vi "SMU tester.vi"() -> ()   [LabVIEW 2021, in "Source meter.lvlib"]
uses:
  Source meter.lvlib
  ctls/SMU settings.ctl
  ctls/SMU status.ctl
  ctls/MSG to SMU.ctl
  ctls/SMU Commands.ctl
  Messenger service/MessengerLib.lvlib
panel:
  out "Event Logger":string[](array[string])
  out "data":dbl
  out "SMU status":T1 {"Measure Function" items=["Volts", "Current", "Auto Resistance", "Manual Resistance", "Digitize Voltage", "Digitize Current"]; "Source Mode" items=["Voltage", "Current"]}
  out "Last msg":timestamp
  out "Last log msg":string
  in  "VISA resource name":refnum<visa-resource-name>
  out "Waveform Chart":dbl(graph)
  in  "Measurement settings":T2={"Source Mode "=1, "Source Level"=0.001, "Source Limit"=0.1, "Measure Function"=0, "Remote sense"=FALSE, "Clear buffer?"=FALSE, "Beep"=FALSE, "High Capacity"=FALSE, "Terminals"=0, "PLCs"=1.0, "Fast measurement"=FALSE} {"Measure Function" items=["Volts", "Current", "Auto Resistance", "Manual Resistance", "Digitize Voltage", "Digitize Current"]; "Source Mode" items=["Voltage", "Current"]; "Terminals" items=["Front", "Rear"]}
  in  "Disconnect":bool
  in  "Setup measuerment":bool
  in  "Start measurment":bool
  in  "Stop measurement":bool
  in  "End":bool
  in  "Connect":bool
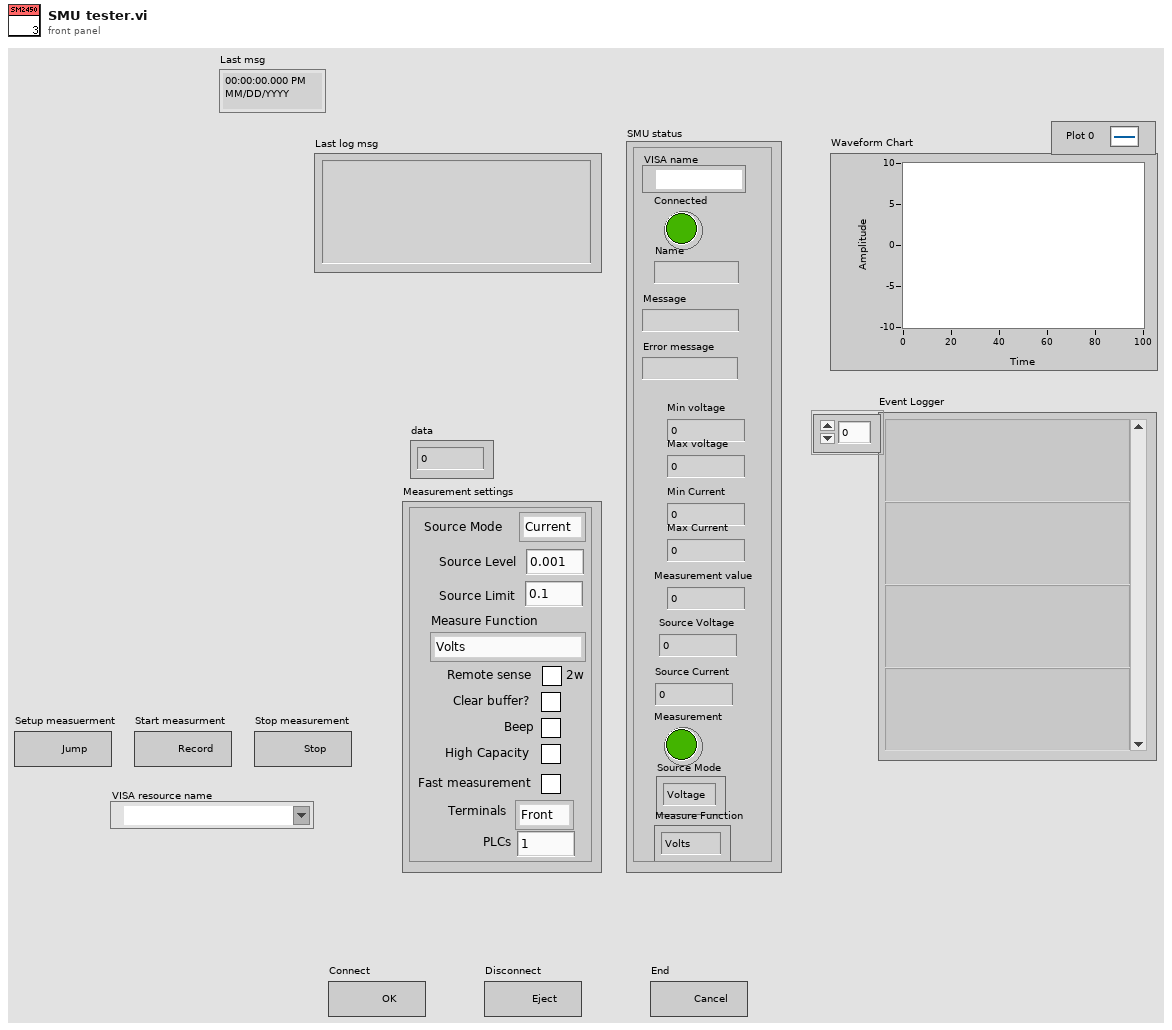
[diagram p1: front panel]
types:
  T1 = typedef "Source meter.lvlib/SMU status.ctl" = cluster{"VISA name":refnum<visa-resource-name>, "Connected":bool, "Name":string, "Message":string, "Error message":string, "Min voltage":dbl, "Max voltage":dbl, "Min Current":dbl, "Max Current":dbl, "Measurement value":dbl, "Source Voltage":dbl, "Measurement":bool, "Source Current":dbl, "Source Mode":u16, "Measure Function":u16}
  T2 = typedef "SMU settings.ctl" = cluster{"Source Mode ":u16, "Source Level":dbl, "Source Limit":dbl, "Measure Function":u16, "Remote sense":bool, "Clear buffer?":bool, "Beep":bool, "High Capacity":bool, "Terminals":u16, "PLCs":dbl, "Fast measurement":bool}
  T3 = enum16{"Initializze", "Wait for event", "Check message", "End"}
  T4 = typedef "Source meter.lvlib/MSG to SMU.ctl" = cluster{"Command":T5, "Data":variant}
  T5 = typedef "Source meter.lvlib/SMU Commands.ctl" = enum16{"Ignore", "Connect", "Update", "Set measurement", "Start measurement", "Get actual results", "Stop measurement", "Disconnect", "End"}
  T6 = typedef "MessengerLib.lvlib/MSG to TOP.ctl" = cluster{"Module":T7, "Response":string, "Data":variant, "Time":timestamp}
  T7 = typedef "Module name.ctl" = enum16{"Emty", "Magnet", "VTI", "Excitation", "Servo", "Acquisition", "Rotator", "Digitizer", "SMU2450", "Carousel", "Multimeter", "Tmp monitor", "Power monitor"}
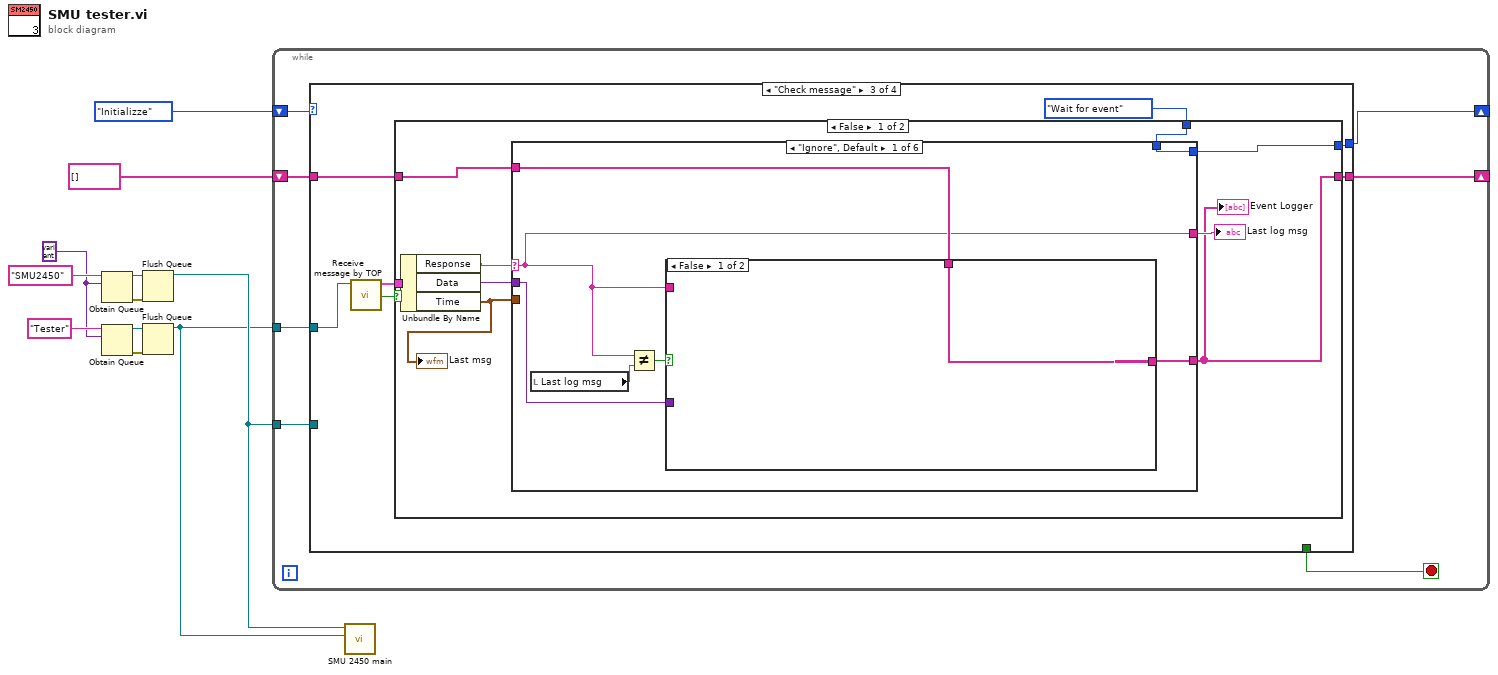
[diagram p0: block diagram]
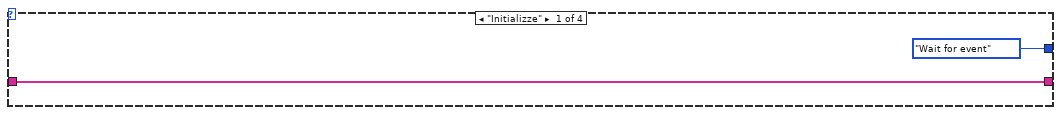
[diagram p2: hidden frame]
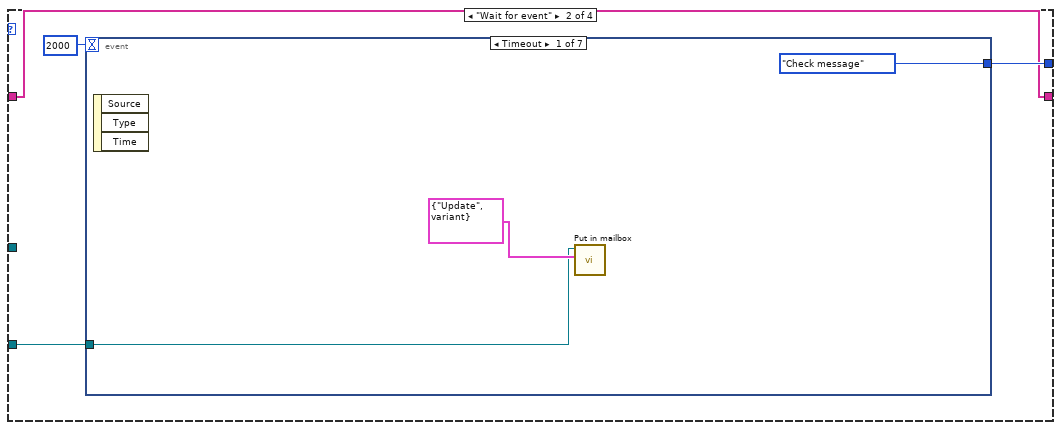
[diagram p3: hidden frame]
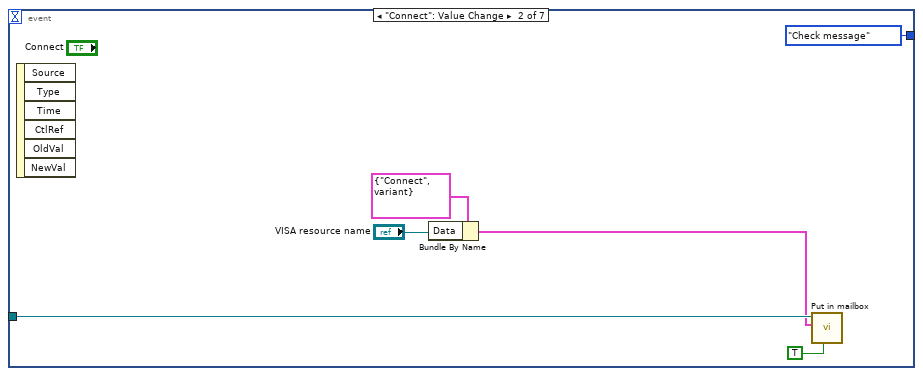
[diagram p4: hidden frame]
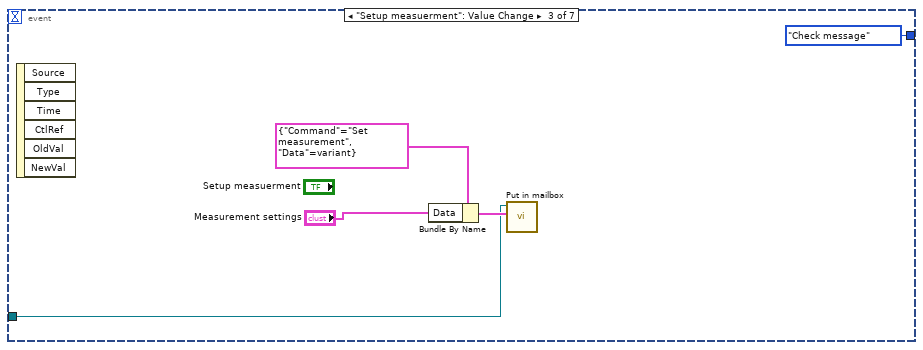
[diagram p5: hidden frame]
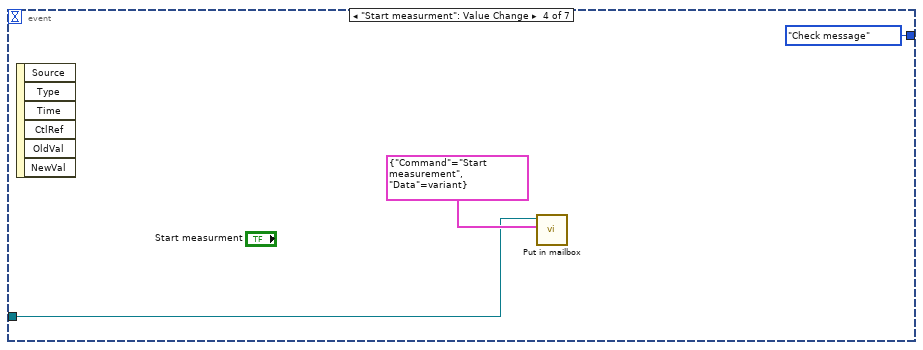
[diagram p6: hidden frame]
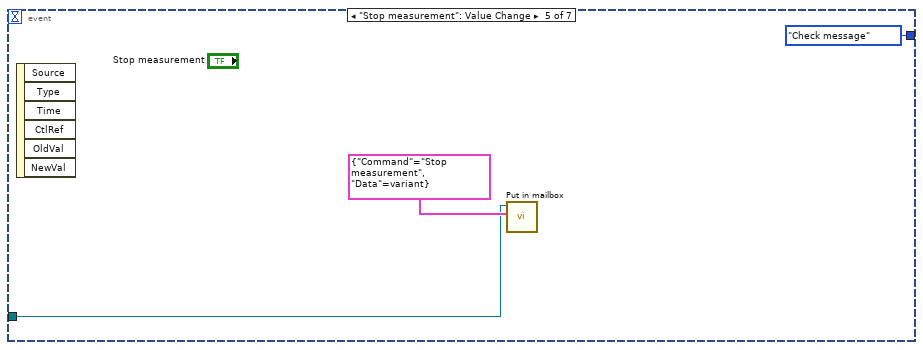
[diagram p7: hidden frame]
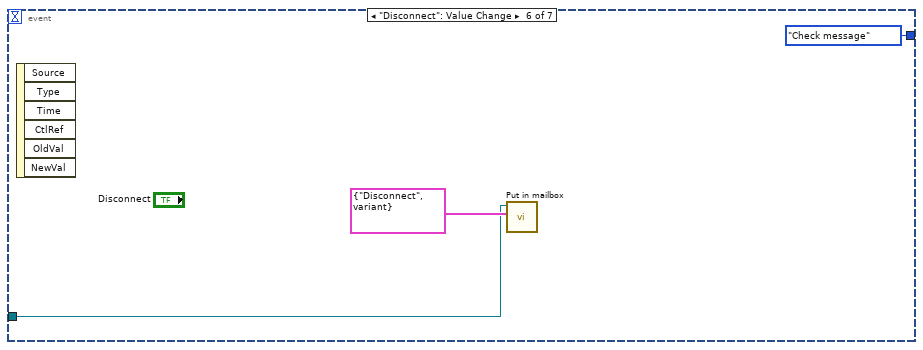
[diagram p8: hidden frame]
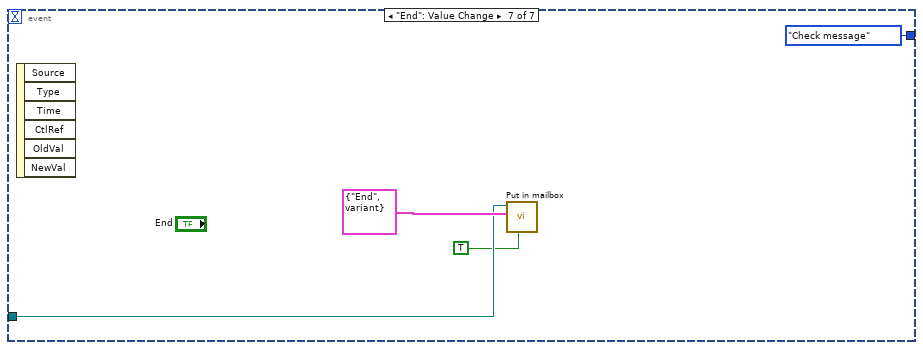
[diagram p9: hidden frame]
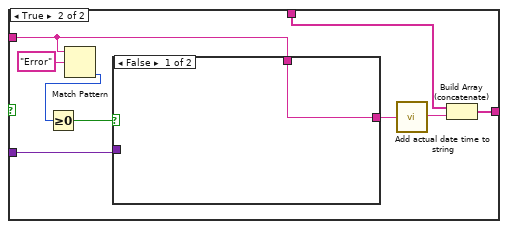
[diagram p10: hidden frame]
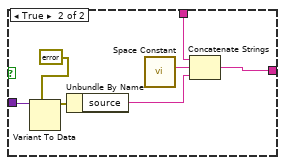
[diagram p11: hidden frame]
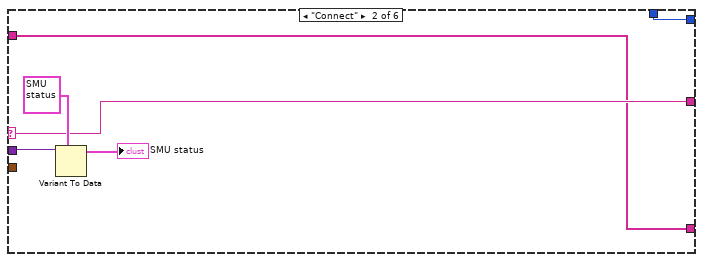
[diagram p12: hidden frame]
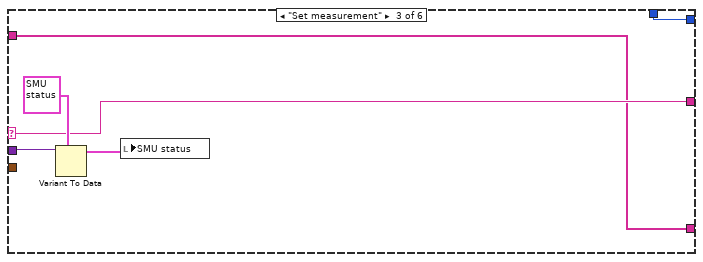
[diagram p13: hidden frame]
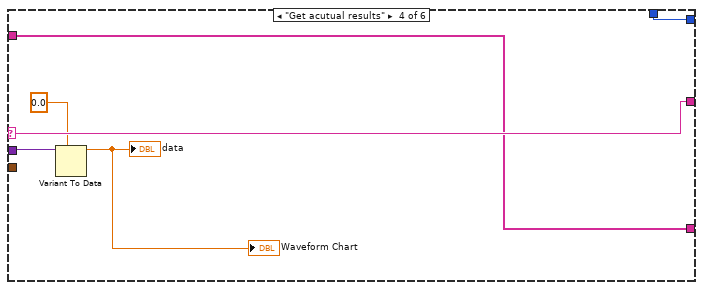
[diagram p14: hidden frame]
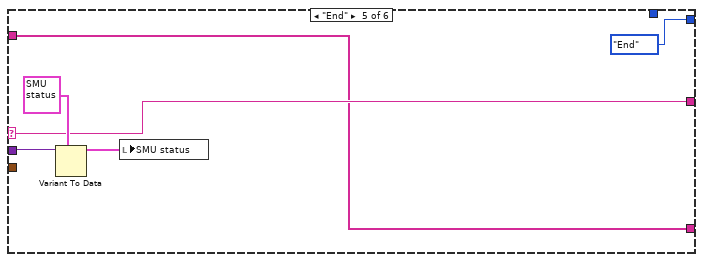
[diagram p15: hidden frame]
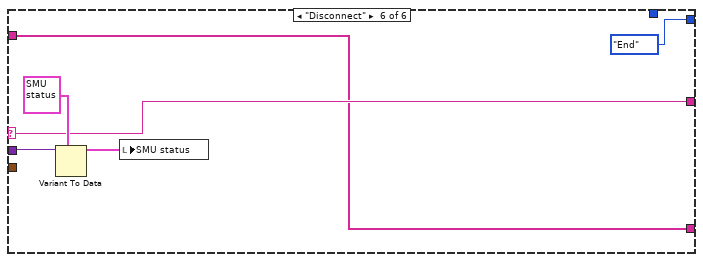
[diagram p16: hidden frame]
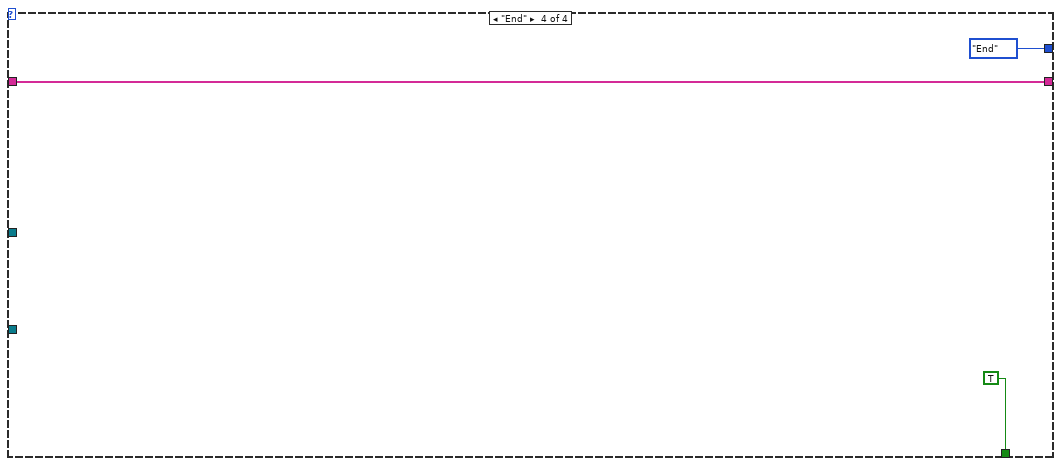
[diagram p18: hidden frame]
diagram:
  w7 = variant
  n1 = Obtain Queue(name (unnamed)="SMU2450", element data type=w7) -> (queue out=w11:refnum<queue>, error out=w5:errorcluster)  [unwired: 3 in, 1 out]
  n2 = Obtain Queue(name (unnamed)="Tester", element data type=w7) -> (queue out=w8:refnum<queue>, error out=w6:errorcluster)  [unwired: 3 in, 1 out]
  n3 = Flush Queue(queue=w11, error in (no error)=w5) -> (queue out=w3:refnum<queue>)  [unwired: 2 out]
  n4 = Flush Queue(queue=w8, error in (no error)=w6) -> (queue out=w2:refnum<queue>)  [unwired: 2 out]
  n5 = while {
    shift-right: [w17] -> _
    shift-left: T3."Initializze" -> [w18]
    tunnel: w3 -> [w16]
    tunnel: w2 -> [w15]
    shift-right: [w12] -> _
    shift-left: string[] [] ("Event Logger") -> [w13]
    stop <- w14 stop-if-true
    n6 = case shown="\"Check message\"" w18 {
      tunnel: [T3."Wait for event" w24 w55 T3."End"] -> w17
      tunnel: w16 -> [_ w23 _ _]
      tunnel: w15 -> [_ _ w58 _]
      tunnel: [_ _ _ TRUE] -> w14
      tunnel: w13 -> [w19 w21 w53 w125]
      tunnel: [w19 w21 w52 w125] -> w12
      frame "Initializze" {
      }
      frame "Wait for event" {
        n7 = event shown="[0] Timeout" {
          selector: _ -> [_ _ _ _ _ _ _]
          dyn-events: _ -> [_ _ _ _ _ _ _]
          timeout: 2000 -> [_ _ _ _ _ _ _]
          tunnel: [T3."Check message" T3."Check message" T3."Check message" T3."Check message" T3."Check message" T3."Check message" T3."Check message"] -> w24
          tunnel: w23 -> [w25 w33 w34 w40 w43 w46 w50]
          event Timeout {
            n8 = event-data() -> ()  [unwired: 1 in, 3 out]
            n9 = call "Put in mailbox.vi"("Message"=T4 {"Command"=enum."Update", "Data"=variant} ("MSG to Source meter"), "Queue in"=w25) -> ()  [unwired: 7 in, 3 out]
          }
          event "Connect": Value Change {
            n10 = event-data() -> ()  [unwired: 1 in, 6 out]
            n11 = Bundle By Name(cluster=T4 {"Command"=enum."Connect", "Data"=variant} ("MSG to Source meter"), "Data"="VISA resource name") -> (w31:T4)
            n12 = call "Put in mailbox.vi"("Priority? (F)"=TRUE, "Message"=w31, "Queue in"=w33) -> ()  [unwired: 6 in, 3 out]
          }
          event "Setup measuerment": Value Change {
            n13 = event-data() -> ()  [unwired: 1 in, 6 out]
            n14 = Bundle By Name(cluster=T4 {"Command"=enum."Set measurement", "Data"=variant} ("MSG to Source meter"), "Data"="Measurement settings") -> (w37:T4)
            n15 = call "Put in mailbox.vi"("Message"=w37, "Queue in"=w34) -> ()  [unwired: 7 in, 3 out]
          }
          event "Start measurment": Value Change {
            n16 = event-data() -> ()  [unwired: 1 in, 6 out]
            n17 = call "Put in mailbox.vi"("Message"=T4 {"Command"=enum."Start measurement", "Data"=variant} ("MSG to Source meter"), "Queue in"=w40) -> ()  [unwired: 7 in, 3 out]
          }
          event "Stop measurement": Value Change {
            n18 = event-data() -> ()  [unwired: 1 in, 6 out]
            n19 = call "Put in mailbox.vi"("Message"=T4 {"Command"=enum."Stop measurement", "Data"=variant} ("MSG to Source meter"), "Queue in"=w43) -> ()  [unwired: 7 in, 3 out]
          }
          event "Disconnect": Value Change {
            n20 = event-data() -> ()  [unwired: 1 in, 6 out]
            n21 = call "Put in mailbox.vi"("Message"=T4 {"Command"=enum."Disconnect", "Data"=variant} ("MSG to Source meter"), "Queue in"=w46) -> ()  [unwired: 7 in, 3 out]
          }
          event "End": Value Change {
            n22 = event-data() -> ()  [unwired: 1 in, 6 out]
            n23 = call "Put in mailbox.vi"("Priority? (F)"=TRUE, "Message"=T4 {"Command"=enum."End", "Data"=variant} ("MSG to Source meter"), "Queue in"=w50) -> ()  [unwired: 6 in, 3 out]
          }
        }
      }
      frame "Check message" {
        n24 = call "Receive message by TOP.vi"("Mailbox in"=w58) -> ("timed out?"=w54:bool, "MSG packet"=w57:T6)  [unwired: 7 in, 2 out]
        n25 = case shown="False" w54 {
          tunnel: w57 -> [w67 _]
          tunnel: T3."Wait for event" -> [w66 w124]
          tunnel: [w65 w124] -> w55
          tunnel: w53 -> [w60 w123]
          tunnel: [w59 w123] -> w52
          frame False {
            n26 = Unbundle By Name(w67) -> ("Response"=w64:string, "Data"=w63:variant, "Time"=w62:timestamp)
            "Last msg" <- w62
            n27 = case shown="\"Ignore\", Default" w64 {
              selector: w64 -> [w69 w94 w101 w108 w112 w118]
              tunnel: w66 -> [w74 w98 w104 w110 _ _]
              tunnel: [w74 w98 w104 w110 T3."End" T3."End"] -> w65
              tunnel: w63 -> [w68 w97 w103 w109 w116 w122]
              tunnel: w62 -> [_ _ _ _ _ _]
              tunnel: [w69 w94 w101 w108 w112 w118] -> w61
              tunnel: w60 -> [w73 w93 w100 w106 w111 w117]
              tunnel: [w72 w93 w100 w106 w111 w117] -> w59
              frame "Ignore", Default {
                n28 = local read "Last log msg"() -> (w70:string)
                n29 = Not Equal?(x=w69, y=w70) -> (x != y?=w71:bool)
                n30 = case shown="False" w71 {
                  tunnel: w73 -> [w75 w83]
                  tunnel: [w75 w84] -> w72
                  tunnel: w69 -> [_ w77]
                  tunnel: w68 -> [_ w78]
                  frame False {
                  }
                  frame True {
                    n31 = Match Pattern(string=w77, regular expression="Error") -> (offset past match=w80:i32)  [unwired: 1 in, 3 out]
                    n32 = Greater Or Equal To 0?(x=w80) -> (x >= 0?=w79:bool)
                    n33 = case shown="False" w79 {
                      tunnel: w78 -> [_ w92]
                      tunnel: w77 -> [w85 w87]
                      tunnel: [w85 w86] -> w76
                      frame False {
                      }
                      frame True {
                        n34 = Variant To Data(type=errorcluster {"status"=FALSE, "code"=0, "source"=""} ("error constant"), Variant=w92) -> (data=w90:errorcluster)  [unwired: 1 in, 1 out]
                        n35 = Unbundle By Name(w90) -> ("source"=w88:string)
                        n36 = call <vilib>:"Space Constant.vi"() -> ("String"=w89:string)
                        n37 = Concatenate Strings(w87, w89, w88) -> (w86:string)
                      }
                    }
                    n38 = call "Add actual date time to string.vi"("String in"=w76) -> ("String out"=w82:string)  [unwired: 4 in]
                    n39 = Build Array (concatenate)(w83, w82) -> (w84:string[])
                  }
                }
              }
              frame "Connect" {
                n40 = Variant To Data(type=T1 {"VISA name"="", "Connected"=FALSE, "Name"="", "Message"="", "Error message"="", "Min voltage"=0.0, "Max voltage"=0.0, "Min Current"=0.0, "Max Current"=0.0, "Measurement value"=0.0, "Source Voltage"=0.0, "Measurement"=FALSE, "Source Current"=0.0, "Source Mode"=0, "Measure Function"=0} ("SMU status"), Variant=w97) -> (data=→"SMU status":T1)  [unwired: 1 in, 1 out]
              }
              frame "Set measurement" {
                n41 = Variant To Data(type=T1 {"VISA name"="", "Connected"=FALSE, "Name"="", "Message"="", "Error message"="", "Min voltage"=0.0, "Max voltage"=0.0, "Min Current"=0.0, "Max Current"=0.0, "Measurement value"=0.0, "Source Voltage"=0.0, "Measurement"=FALSE, "Source Current"=0.0, "Source Mode"=0, "Measure Function"=0} ("SMU status"), Variant=w103) -> (data=w99:T1)  [unwired: 1 in, 1 out]
                n42 = local write "SMU status"(w99) -> ()
              }
              frame "Get acutual results" {
                n43 = Variant To Data(type=0.0, Variant=w109) -> (data=→"data" →"Waveform Chart":dbl)  [unwired: 1 in, 1 out]
              }
              frame "End" {
                n44 = Variant To Data(type=T1 {"VISA name"="", "Connected"=FALSE, "Name"="", "Message"="", "Error message"="", "Min voltage"=0.0, "Max voltage"=0.0, "Min Current"=0.0, "Max Current"=0.0, "Measurement value"=0.0, "Source Voltage"=0.0, "Measurement"=FALSE, "Source Current"=0.0, "Source Mode"=0, "Measure Function"=0} ("SMU status"), Variant=w116) -> (data=w114:T1)  [unwired: 1 in, 1 out]
                n45 = local write "SMU status"(w114) -> ()
              }
              frame "Disconnect" {
                n46 = Variant To Data(type=T1 {"VISA name"="", "Connected"=FALSE, "Name"="", "Message"="", "Error message"="", "Min voltage"=0.0, "Max voltage"=0.0, "Min Current"=0.0, "Max Current"=0.0, "Measurement value"=0.0, "Source Voltage"=0.0, "Measurement"=FALSE, "Source Current"=0.0, "Source Mode"=0, "Measure Function"=0} ("SMU status"), Variant=w122) -> (data=w120:T1)  [unwired: 1 in, 1 out]
                n47 = local write "SMU status"(w120) -> ()
              }
            }
            "Last log msg" <- w61
            "Event Logger" <- w59
          }
          frame True {
          }
        }
      }
      frame "End" {
      }
    }
  }
  n48 = call "SMU 2450 main.vi"("Mailbox address Top"=w2, "Module mailbox"=w3) -> ()  [unwired: 8 in, 2 out]
